vi "lxw strerror.vi"(8 "error in (no error)":errorcluster, 11 "error_num":u32(ring) items=["LXW_NO_ERROR", "LXW_ERROR_MEMORY_MALLOC_FAILED", "LXW_ERROR_CREATING_XLSX_FILE", "LXW_ERROR_CREATING_TMPFILE", "LXW_ERROR_READING_TMPFILE", "LXW_ERROR_ZIP_FILE_OPERATION", "LXW_ERROR_ZIP_PARAMETER_ERROR", "LXW_ERROR_ZIP_BAD_ZIP_FILE", "LXW_ERROR_ZIP_INTERNAL_ERROR", "LXW_ERROR_ZIP_FILE_ADD", "LXW_ERROR_ZIP_CLOSE", "LXW_ERROR_FEATURE_NOT_SUPPORTED", "LXW_ERROR_NULL_PARAMETER_IGNORED", "LXW_ERROR_PARAMETER_VALIDATION", "LXW_ERROR_PARAMETER_IS_EMPTY", "LXW_ERROR_SHEETNAME_LENGTH_EXCEEDED", "LXW_ERROR_INVALID_SHEETNAME_CHARACTER", "LXW_ERROR_SHEETNAME_START_END_APOSTROPHE", "LXW_ERROR_SHEETNAME_ALREADY_USED", "LXW_ERROR_32_STRING_LENGTH_EXCEEDED", "LXW_ERROR_128_STRING_LENGTH_EXCEEDED", "LXW_ERROR_255_STRING_LENGTH_EXCEEDED", "LXW_ERROR_MAX_STRING_LENGTH_EXCEEDED", "LXW_ERROR_SHARED_STRING_INDEX_NOT_FOUND", "LXW_ERROR_WORKSHEET_INDEX_OUT_OF_RANGE", "LXW_ERROR_WORKSHEET_MAX_URL_LENGTH_EXCEEDED", "LXW_ERROR_WORKSHEET_MAX_NUMBER_URLS_EXCEEDED", "LXW_ERROR_IMAGE_DIMENSIONS"]) -> (0 "error out":errorcluster, 3 "function return":string)   [LabVIEW 8.6]
doc: "char* lxw_strerror(lxw_error error_num);"
uses:
  pending_lvxlsxwriter/xlsxwriter.dll
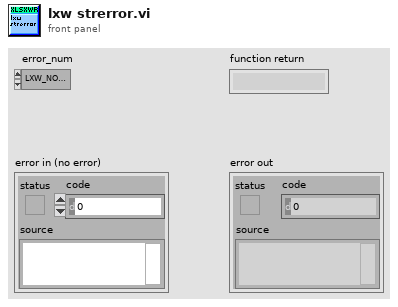
[diagram p1: front panel]
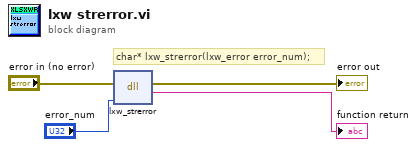
[diagram p0: block diagram]
diagram:
  # "char* lxw_strerror(lxw_error error_num);"
  n1 = dll-call lib="C:/Users/WDAGUtilityAccount/Desktop/pending_lvxlsxwriter/xlsxwriter.*" fn="lxw_strerror"(error in="error in (no error)", "error_num"="error_num") -> (error out=→"error out":errorcluster, →"function return":string)  [unwired: 3 in, 1 out]
